vi "CloseSail.vi"(8 "error in (no error)":errorcluster, 11 "RealSail in":refnum<class "RealSail.lvclass">) -> (0 "error out":errorcluster, 3 "RealSail out":refnum<class "RealSail.lvclass">)   [LabVIEW 2013, in "RealSail.lvclass"]
uses:
  RealSail.lvclass
  AbstractSail/AbstractSail.lvclass
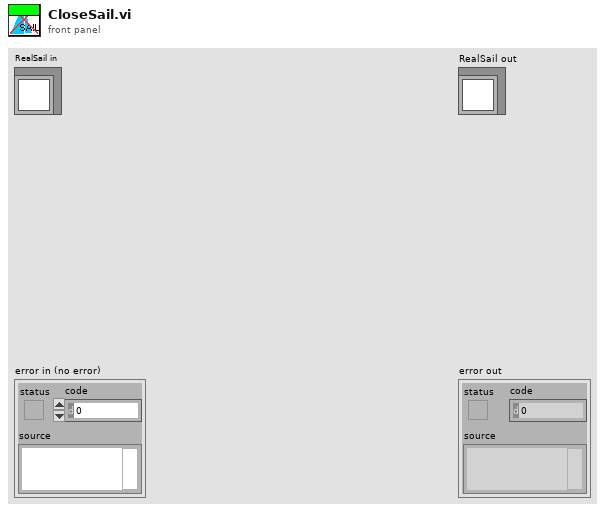
[diagram p1: front panel]
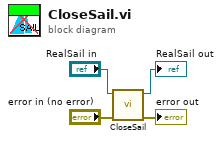
[diagram p0: block diagram]
diagram:
  n1 = call-parent "CloseSail.vi"("error in (no error)"="error in (no error)", "AbstractSail in"="RealSail in") -> ("error out"=→"error out":errorcluster, "AbstractSail out"=→"RealSail out":refnum<class "RealSail.lvclass">)  [unwired: 8 in]
